vi "Python DENSO Communication.vi"() -> ()   [LabVIEW 2022 SP3]
uses:
  <vilib>/ImagingLab/Denso Robotics Library/_Private/Controls/drl_Variable T.ctl
  <vilib>/ImagingLab/Denso Robotics Library/_Private/Controls/drl_Motion parameters.ctl
  <vilib>/ImagingLab/Denso Robotics Library/_Private/Controls/drl_Interpolation.ctl
  <vilib>/ImagingLab/Denso Robotics Library/_Private/Controls/drl_Pass motion.ctl
  <vilib>/ImagingLab/Denso Robotics Library/_Private/Controls/drl_Move option.ctl
  <vilib>/ImagingLab/Denso Robotics Library/_Private/Controls/drl_Robot Coordinates.ctl
  <vilib>/ImagingLab/Denso Robotics Library/_Private/Controls/drl_Variable J.ctl
  <vilib>/Utility/error.llb/DialogType.ctl
  <vilib>/addons/zeromq/socket_type.ctl
  <vilib>/ImagingLab/Denso Robotics Library/_Private/Controls/drl_Robot Session.ctl
  <vilib>/ImagingLab/Denso Robotics Library/_Private/Controls/drl_Open Data.ctl
  <vilib>/ImagingLab/Denso Robotics Library/_Private/Controls/drl_Controller_IP Address.ctl
  <vilib>/ImagingLab/Denso Robotics Library/_Private/Controls/drl_Robot type.ctl
  <vilib>/ImagingLab/Denso Robotics Library/_Private/Controls/drl_controller_type.ctl
  <vilib>/ImagingLab/Denso Robotics Library/_Private/Controls/drl_Robot Motor status.ctl
  <vilib>/ImagingLab/Denso Robotics Library/_Private/Controls/drl_RobSlave actions.ctl
  <vilib>/ImagingLab/Denso Robotics Library/_Private/Controls/drl_Get_Set.ctl
  <vilib>/ImagingLab/Denso Robotics Library/_Private/Controls/drl_TOOL.ctl
  <vilib>/ImagingLab/Denso Robotics Library/_Public/SubVIs/drl_Robot Move_TRANS.vi
  <vilib>/ImagingLab/Denso Robotics Library/_Public/SubVIs/drl_Robot Move_JOINT.vi
  <vilib>/ImagingLab/Denso Robotics Library/_Public/SubVIs/drl_Robot Move_CARTESIAN.vi
  <vilib>/ImagingLab/Denso Robotics Library/_Public/SubVIs/drl_Get_Robot Angle_J.vi
  <vilib>/ImagingLab/Denso Robotics Library/_Public/SubVIs/drl_Get_Robot Position_P.vi
  <vilib>/ImagingLab/Denso Robotics Library/_Public/SubVIs/drl_Get_Robot Trans_T.vi
  <vilib>/addons/zeromq/zmq_context.lvclass
  <vilib>/addons/zeromq/zmq_socket.lvclass
  <vilib>/addons/zeromq/zeromq.lvlib
  <vilib>/ImagingLab/Denso Robotics Library/DensoRoboticsLibrary.lvlib
panel:
  in  "stop":bool
  in  "Communication port":string="5555"
  out "Motion parameters J":T1
  out "Position J":T5 {"Axis 6" format="%.4f"; "Axis 5" format="%.4f"; "Axis 4" format="%.4f"; "Axis 3" format="%.4f"; "Axis 2" format="%.4f"; "Axis 1" format="%.4f"}
  out "Motion parameters C":T1
  out "Position C":T6 {"X" format="%.4f"; "Y" format="%.4f"; "Z" format="%.4f"; "Rx" format="%.4f"; "Ry" format="%.4f"; "Rz" format="%.4f"}
  out "Motion parameters T":T1
  out "Position T":T7 {"Az" format="%.4f"; "Ay" format="%.4f"; "Ax" format="%.4f"; "Oz" format="%.4f"; "Oy" format="%.4f"; "Ox" format="%.4f"; "Z" format="%.4f"; "Y" format="%.4f"; "X" format="%.4f"}
  out "Message history":string[][](array[string])
  out "Python message string - data":string
  out "Python message string - command":string
  out "Python message string":string
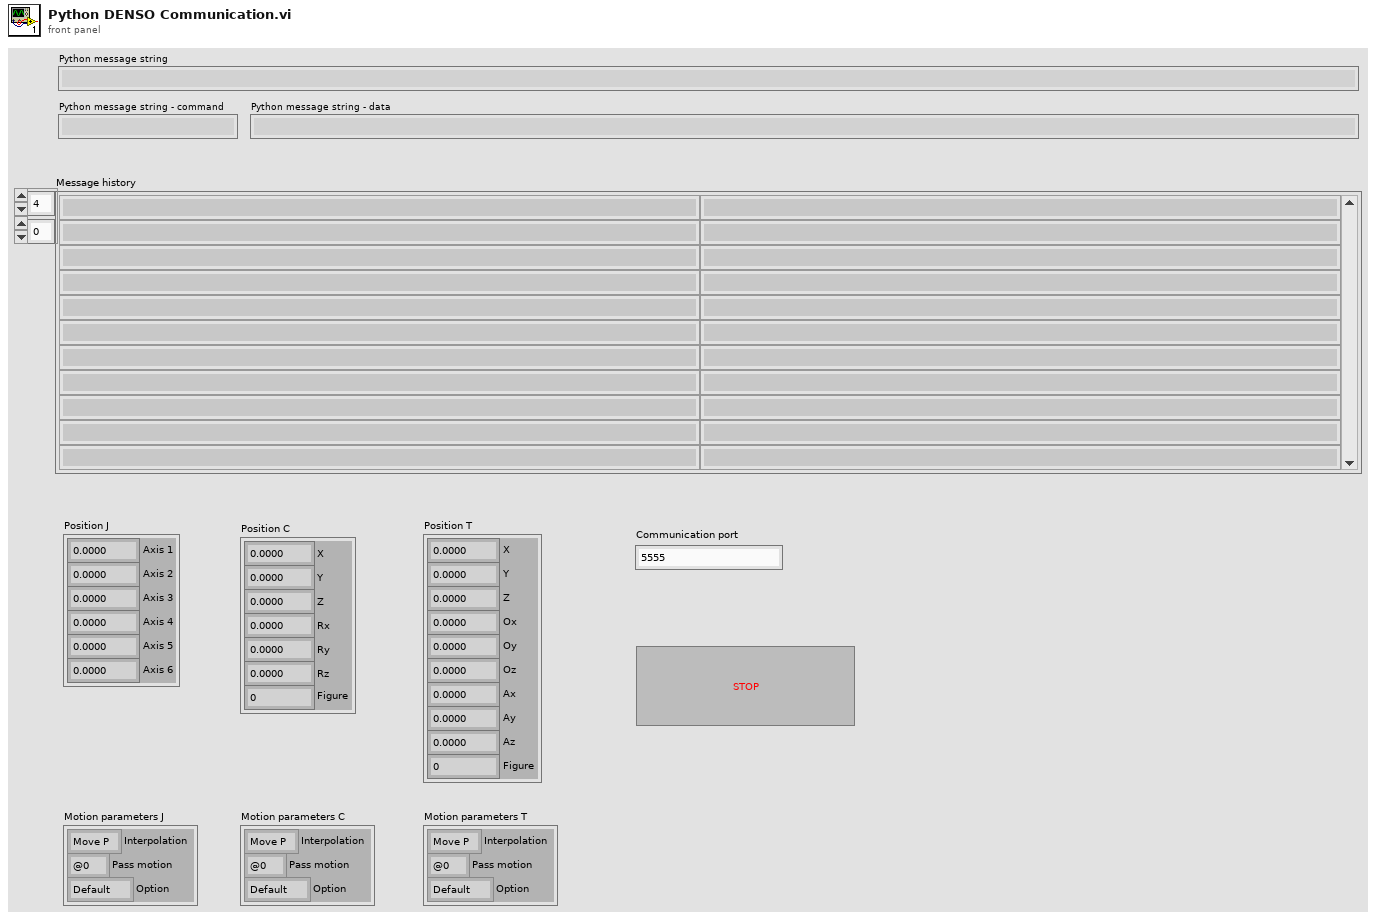
[diagram p1: front panel]
types:
  T1 = typedef "DensoRoboticsLibrary.lvlib/drl_Motion parameters.ctl" = cluster{"Interpolation":T2, "Pass motion":T3, "Option":T4}
  T2 = typedef "DensoRoboticsLibrary.lvlib/drl_Interpolation.ctl" = enum16{"Move P", "Move L"}
  T3 = typedef "DensoRoboticsLibrary.lvlib/drl_Pass motion.ctl" = enum16{"@0", "@P", "@E"}
  T4 = typedef "DensoRoboticsLibrary.lvlib/drl_Move option.ctl" = enum16{"Default", "Next"}
  T5 = typedef "DensoRoboticsLibrary.lvlib/drl_Variable J.ctl" = cluster{"Axis 1":sgl, "Axis 2":sgl, "Axis 3":sgl, "Axis 4":sgl, "Axis 5":sgl, "Axis 6":sgl}
  T6 = typedef "DensoRoboticsLibrary.lvlib/drl_Robot Coordinates.ctl" = cluster{"X":dbl, "Y":dbl, "Z":dbl, "Rx":dbl, "Ry":dbl, "Rz":dbl, "Figure":dbl}
  T7 = typedef "DensoRoboticsLibrary.lvlib/drl_Variable T.ctl" = cluster{"X":sgl, "Y":sgl, "Z":sgl, "Ox":sgl, "Oy":sgl, "Oz":sgl, "Ax":sgl, "Ay":sgl, "Az":sgl, "Figure":sgl}
  T8 = typedef "zeromq.lvlib/socket_type.ctl" = enum8{"ZMQ_PAIR", "ZMQ_PUB", "ZMQ_SUB", "ZMQ_REQ", "ZMQ_REP", "ZMQ_DEALER", "ZMQ_ROUTER", "ZMQ_PULL", "ZMQ_PUSH", "ZMQ_XPUB", "ZMQ_XSUB", "ZMQ_STREAM", "ZMQ_SERVER", "ZMQ_CLIENT", "ZMQ_RADIO", "ZMQ_DISH", "ZMQ_GATHER", "ZMQ_SCATTER", "ZMQ_DGRAM"}
  T9 = typedef "DensoRoboticsLibrary.lvlib/drl_Robot Session.ctl" = string
  T10 = typedef "DensoRoboticsLibrary.lvlib/drl_Open Data.ctl" = cluster{"controller IP address":T11, "robot type":T12, "controller type":T13}
  T11 = typedef "DensoRoboticsLibrary.lvlib/drl_Controller_IP Address.ctl" = string
  T12 = typedef "DensoRoboticsLibrary.lvlib/drl_Robot type.ctl" = enum16{"6 axes", "5 axes", "4 axes"}
  T13 = typedef "DensoRoboticsLibrary.lvlib/drl_controller_type.ctl" = enum16{"RC7", "RC8"}
  T14 = typedef "DensoRoboticsLibrary.lvlib/drl_Robot Motor status.ctl" = enum16{"Motor OFF", "Motor ON"}
  T15 = typedef "DensoRoboticsLibrary.lvlib/drl_RobSlave actions.ctl" = enum16{"Start", "Stop"}
  T16 = typedef "DensoRoboticsLibrary.lvlib/drl_Get_Set.ctl" = enum16{"Get", "Set"}
  T17 = typedef "DensoRoboticsLibrary.lvlib/drl_TOOL.ctl" = cluster{"X":sgl, "Y":sgl, "Z":sgl, "RX":sgl, "RY":sgl, "RZ":sgl}
  T18 = typedef "DialogType.ctl" = u16
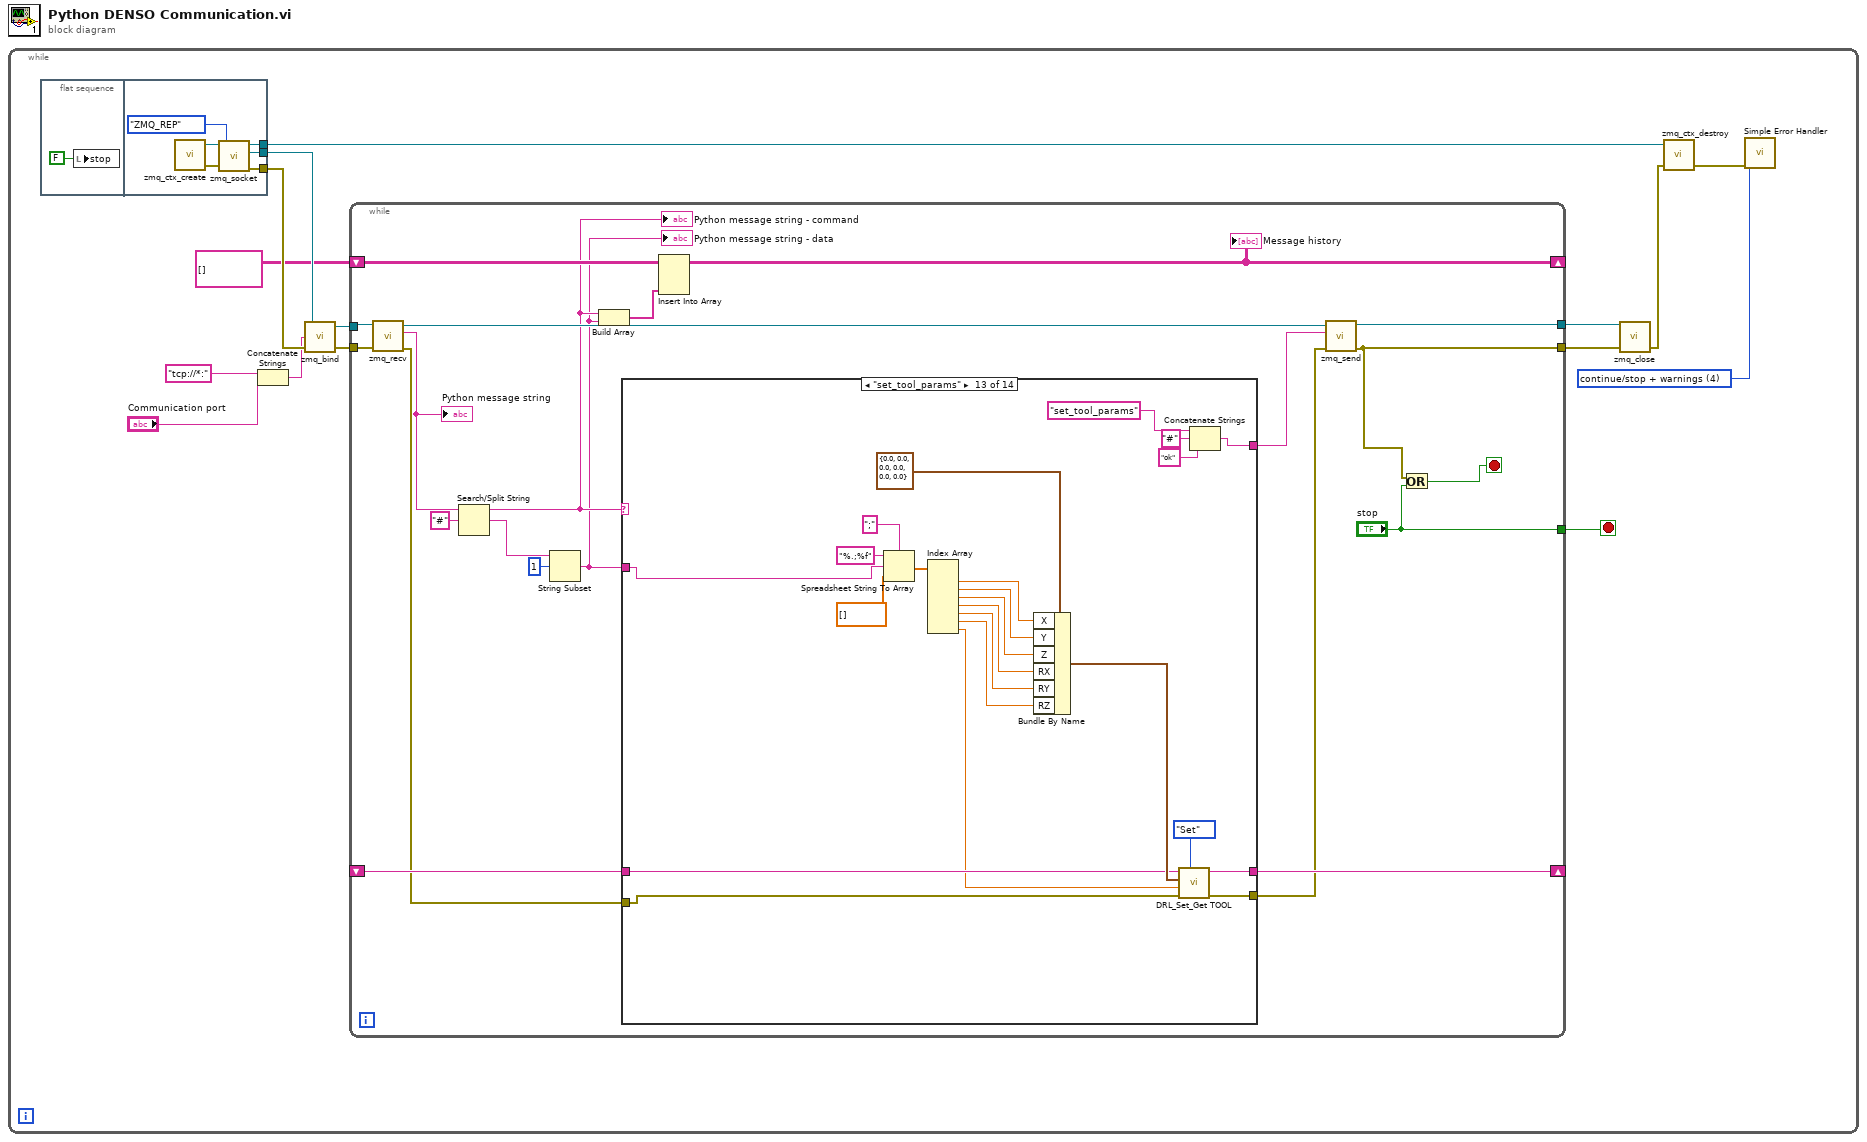
[diagram p0: block diagram]
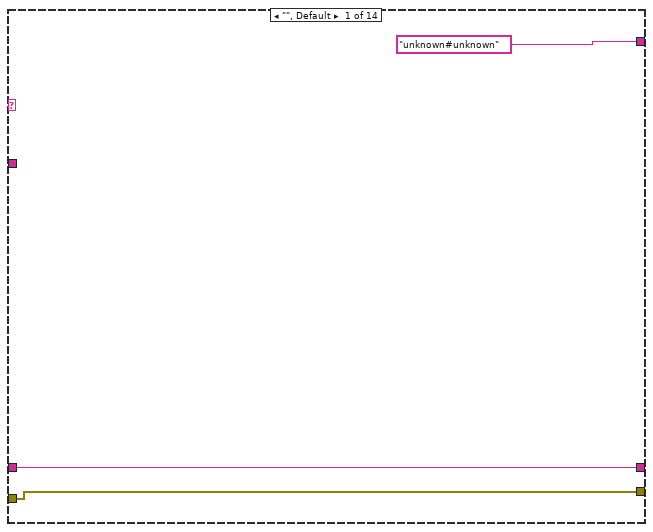
[diagram p2: hidden frame]
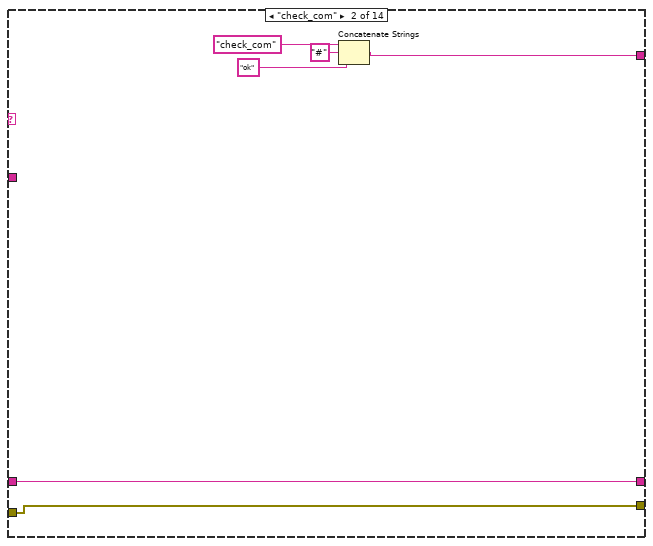
[diagram p3: hidden frame]
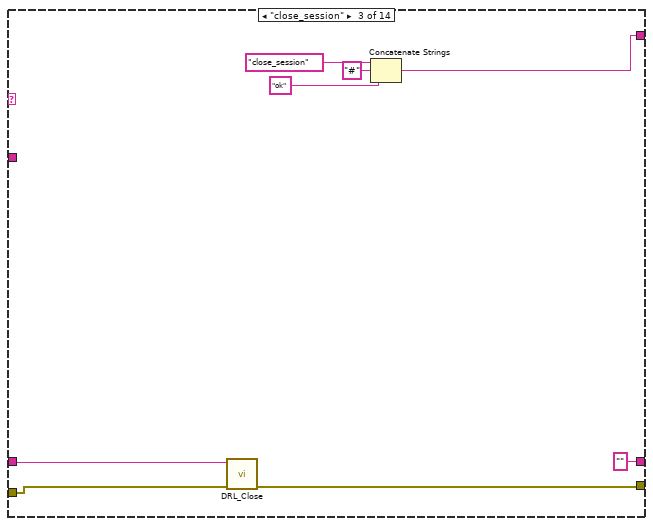
[diagram p4: hidden frame]
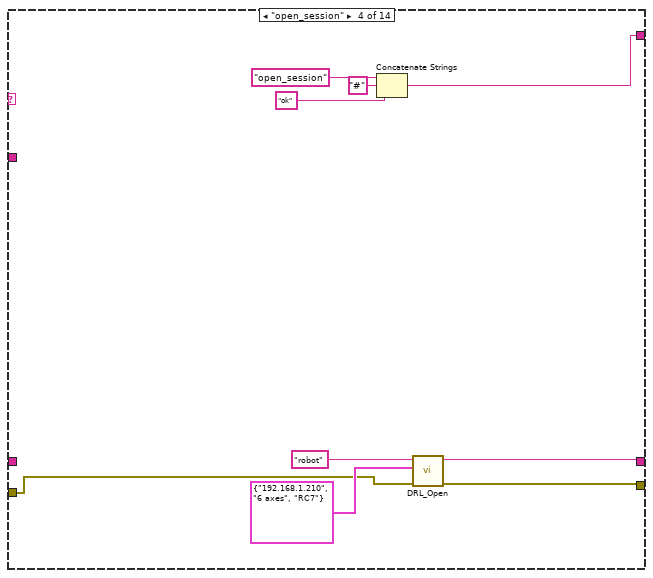
[diagram p5: hidden frame]
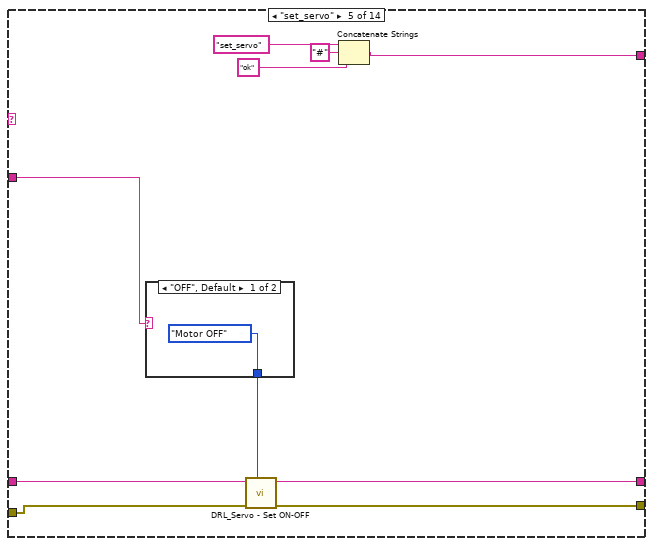
[diagram p6: hidden frame]
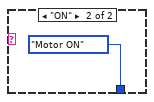
[diagram p7: hidden frame]
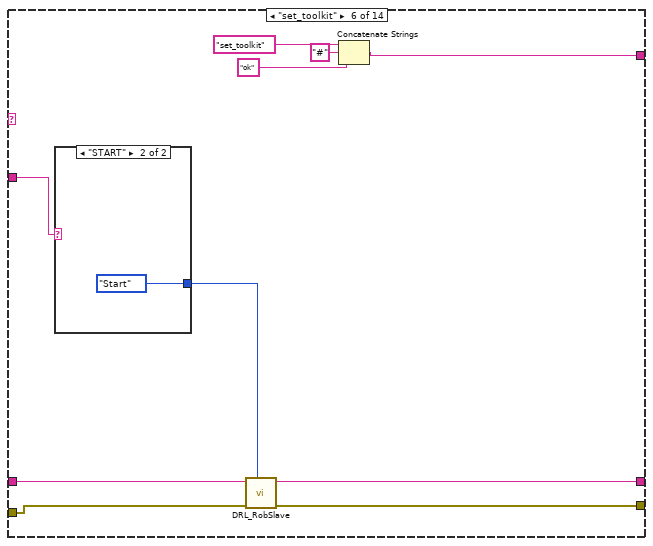
[diagram p8: hidden frame]
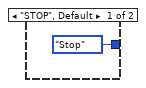
[diagram p9: hidden frame]
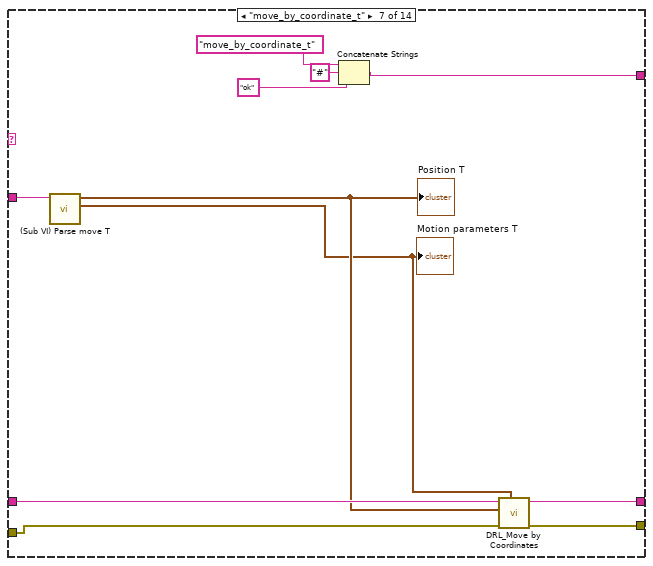
[diagram p10: hidden frame]
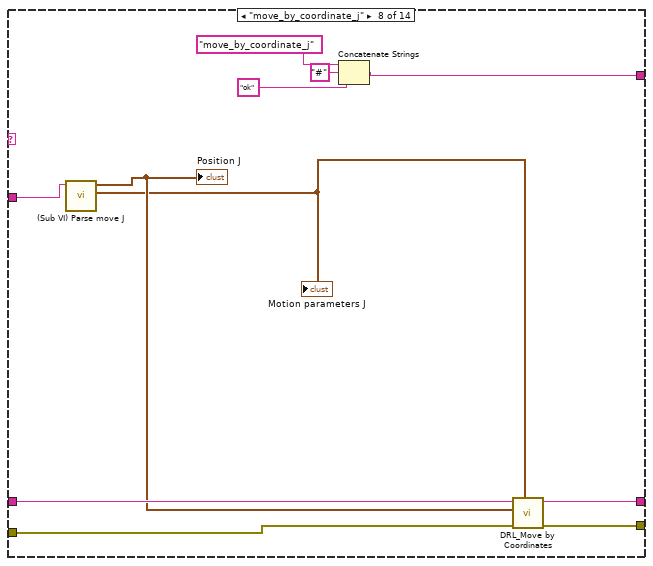
[diagram p11: hidden frame]
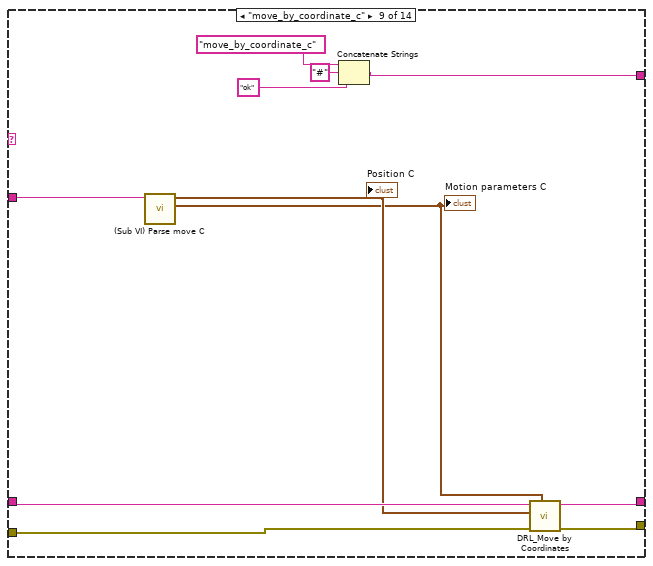
[diagram p12: hidden frame]
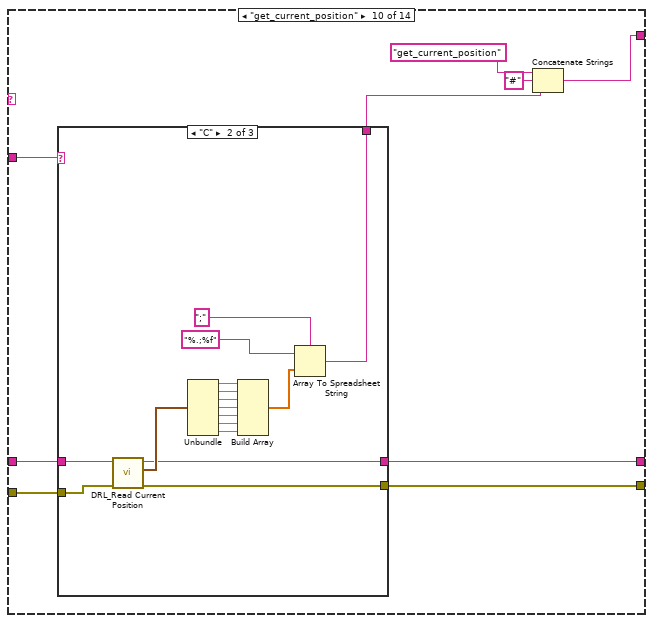
[diagram p13: hidden frame]
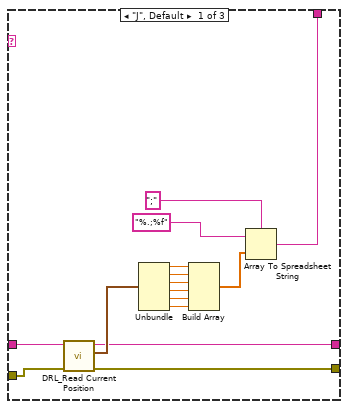
[diagram p14: hidden frame]
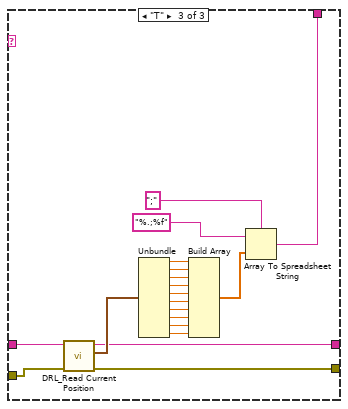
[diagram p15: hidden frame]
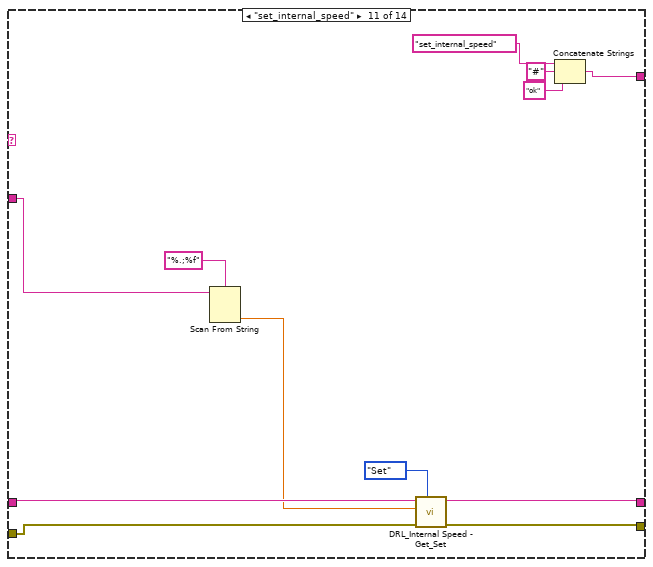
[diagram p16: hidden frame]
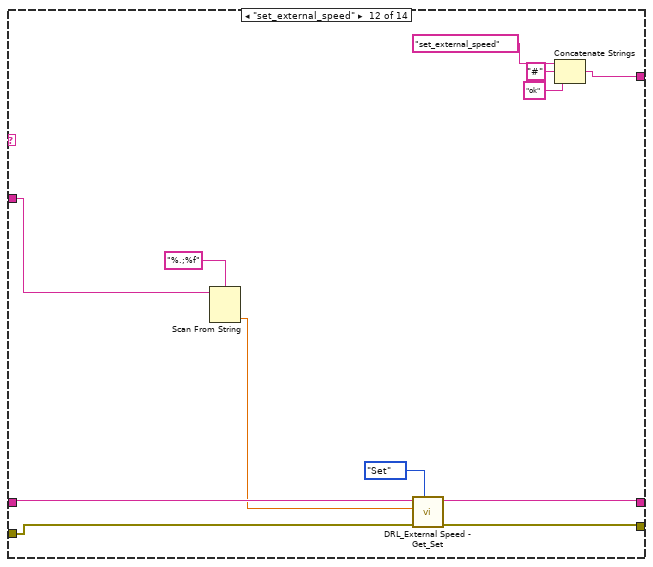
[diagram p17: hidden frame]
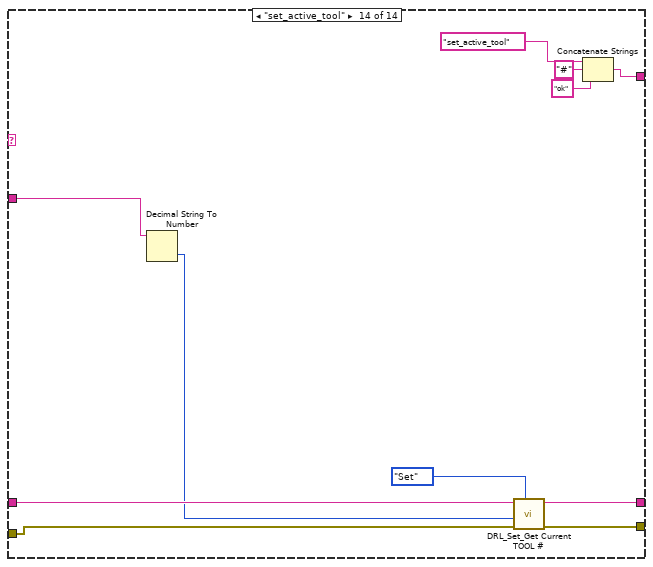
[diagram p18: hidden frame]
diagram:
  n1 = while {
    stop <- w1 stop-if-true
    w2 = T18 4 items=["no dialog", "OK message", "continue or stop message", "OK message + warnings", "continue/stop + warnings"] ("type of dialog (OK msg:1)")
    n2 = flat-sequence {
      tunnel: [w22] -> w15
      tunnel: [w21] -> w14
      tunnel: [w17] -> w8
      frame #0 {
        n3 = local write "stop"(FALSE ("stop")) -> ()
      }
      frame #1 {
        n4 = call <vilib>:"zmq_ctx_create.vi"() -> ("error out"=w20:errorcluster, "context out"=w19:refnum<class "zmq_context.lvclass">)  [unwired: 4 in]
        n5 = call <vilib>:"zmq_socket.vi"("error in"=w20, "socket type"=socket_type."ZMQ_REP", "context in"=w19) -> ("error out"=w22:errorcluster, "socket out"=w21:refnum<class "zmq_socket.lvclass">, "context out"=w17:refnum<class "zmq_context.lvclass">)  [unwired: 2 in]
      }
    }
    n6 = Concatenate Strings("tcp://*:" ("endpoint"), "Communication port") -> (w4:string)
    n7 = call <vilib>:"zmq_bind.vi"("error in"=w15, "endpoint"=w4, "socket in"=w14) -> ("error out"=w12:errorcluster, "socket out"=w13:refnum<class "zmq_socket.lvclass">)  [unwired: 1 in]
    n8 = while {
      tunnel: w13 -> [w42]
      tunnel: w12 -> [w43]
      tunnel: [w25] -> w11
      tunnel: [w40] -> w10
      shift-right: [w33] -> _
      shift-left: string[][] [] -> [w34]
      shift-right: [w29] -> _
      shift-left: _ -> [w28]
      tunnel: ["stop"] -> w1
      stop <- w24 stop-if-true
      n9 = call <vilib>:"zmq_recv.vi"("error in"=w43, "socket in"=w42) -> ("error out"=w27:errorcluster, "data"=w39:string, "socket out"=w41:refnum<class "zmq_socket.lvclass">)  [unwired: 3 in, 2 out]
      "Python message string" <- w39
      n10 = Search/Split String(string=w39, search string/char (-)="#") -> (substring before match=w32:string, match + rest of string=w37:string)  [unwired: 1 in, 1 out]
      "Python message string - command" <- w32
      n11 = String Subset(string=w37, offset (0)=1) -> (substring=w31:string)  [unwired: 1 in]
      "Python message string - data" <- w31
      n12 = Build Array(w32, w31) -> (w30:string[])
      n13 = case shown="\"set_tool_params\"" w32 {
        tunnel: w31 -> [_ _ _ _ w72 w85 w100 w111 w122 w135 w193 w205 w210 w240]
        tunnel: ["unknown#unknown" w49 w55 w63 w76 w88 w101 w112 w123 w131 w194 w206 w213 w235] -> w35
        tunnel: [w45 w48 T9 "" ("robot session*") w67 w73 w86 w96 w107 w118 w130 w188 w202 w219 w241] -> w29
        tunnel: w28 -> [w45 w48 w60 _ w74 w87 w99 w110 w121 w134 w191 w203 w218 w242]
        tunnel: w27 -> [w44 w47 w54 w62 w71 w83 w95 w106 w116 w128 w187 w199 w212 w234]
        tunnel: [w44 w47 w53 w61 w70 w82 w94 w105 w117 w127 w186 w198 w211 w233] -> w26
        frame "", Default {
        }
        frame "check_com" {
          n14 = Concatenate Strings("check_com", "#" ("string"), "ok" ("string")) -> (w49:string)
        }
        frame "close_session" {
          n15 = call <vilib>:"DRL_Close.vi"("error in (no error)"=w54, "robot session"=w60) -> ("error out"=w53:errorcluster)  [unwired: 9 in]
          n16 = Concatenate Strings("close_session", "#" ("string"), "ok" ("string")) -> (w55:string)
        }
        frame "open_session" {
          n17 = Concatenate Strings("open_session", "#" ("string"), "ok" ("string")) -> (w63:string)
          n18 = call <vilib>:"DRL_Open.vi"("error in (no error)"=w62, "connection settings"=T10 {"controller IP address"="192.168.1.210", "robot type"=enum."6 axes", "controller type"=enum."RC7"}, "robot session"=T9 "robot") -> ("error out"=w61:errorcluster, "robot session*"=w67:T9)  [unwired: 7 in]
        }
        frame "set_servo" {
          n19 = case shown="\"OFF\", Default" w72 {
            tunnel: [drl_Robot_Motor_status."Motor OFF" ("servo status") drl_Robot_Motor_status."Motor ON" ("servo status")] -> w75
            frame "OFF", Default {
            }
            frame "ON" {
            }
          }
          n20 = call <vilib>:"DRL_Servo - Set ON-OFF.vi"("servo status"=w75, "error in (no error)"=w71, "robot session"=w74) -> ("error out"=w70:errorcluster, "robot session*"=w73:T9)  [unwired: 7 in]
          n21 = Concatenate Strings("set_servo", "#" ("string"), "ok" ("string")) -> (w76:string)
        }
        frame "set_toolkit" {
          n22 = case shown="\"START\"" w85 {
            tunnel: [drl_RobSlave_actions."Stop" ("action") drl_RobSlave_actions."Start" ("action")] -> w84
            frame "STOP", Default {
            }
            frame "START" {
            }
          }
          n23 = call <vilib>:"DRL_RobSlave.vi"("action"=w84, "error in (no error)"=w83, "robot session"=w87) -> ("error out"=w82:errorcluster, "robot session*"=w86:T9)  [unwired: 7 in]
          n24 = Concatenate Strings("set_toolkit", "#" ("string"), "ok" ("string")) -> (w88:string)
        }
        frame "move_by_coordinate_t" {
          n25 = call "(Sub VI) Parse move T.vi"("data"=w100) -> ("Motion parameters"=w97:T1, "Position T"=w98:T7)  [unwired: 9 in]
          "Position T" <- w98
          "Motion parameters T" <- w97
          n26 = Concatenate Strings("move_by_coordinate_t", "#" ("string"), "ok" ("string")) -> (w101:string)
          n27 = call-poly <vilib>:"DRL_Move by Coordinates.vi"("motion parameters"=w97, "error in (no error)"=w95, "position T"=w98, "robot session"=w99) -> ("error out"=w94:errorcluster, "robot session*"=w96:T9)  [unwired: 6 in]
        }
        frame "move_by_coordinate_j" {
          n28 = call "(Sub VI) Parse move J.vi"("data"=w111) -> ("Motion parameters"=w108:T1, "Position J"=w109:T5)  [unwired: 9 in]
          "Position J" <- w109
          "Motion parameters J" <- w108
          n29 = Concatenate Strings("move_by_coordinate_j", "#" ("string"), "ok" ("string")) -> (w112:string)
          n30 = call-poly <vilib>:"DRL_Move by Coordinates.vi"("motion parameters"=w108, "error in (no error)"=w106, "position J"=w109, "robot session"=w110) -> ("error out"=w105:errorcluster, "robot session*"=w107:T9)  [unwired: 6 in]
        }
        frame "move_by_coordinate_c" {
          n31 = call "(Sub VI) Parse move C.vi"("data"=w122) -> ("Motion parameters"=w119:T1, "Position C"=w120:T6)  [unwired: 9 in]
          "Position C" <- w120
          "Motion parameters C" <- w119
          n32 = Concatenate Strings("move_by_coordinate_c", "#" ("string"), "ok" ("string")) -> (w123:string)
          n33 = call-poly <vilib>:"DRL_Move by Coordinates.vi"("motion parameters"=w119, "error in (no error)"=w116, "robot coordinates"=w120, "robot session"=w121) -> ("error out"=w117:errorcluster, "robot session*"=w118:T9)  [unwired: 6 in]
        }
        frame "get_current_position" {
          n34 = case shown="\"C\"" w135 {
            tunnel: w134 -> [w150 w166 w185]
            tunnel: [w148 w164 w183] -> w130
            tunnel: [w138 w154 w173] -> w129
            tunnel: w128 -> [w137 w152 w168]
            tunnel: [w136 w151 w167] -> w127
            frame "J", Default {
              n35 = call-poly <vilib>:"DRL_Read Current Position.vi"("error in (no error)"=w137, "robot session"=w150) -> ("error out"=w136:errorcluster, "position J"=w149:T5, "robot session*"=w148:T9)  [unwired: 7 in]
              n36 = Unbundle(w149) -> ("Axis 1"=w145:sgl, "Axis 2"=w144:sgl, "Axis 3"=w143:sgl, "Axis 4"=w142:sgl, "Axis 5"=w141:sgl, "Axis 6"=w140:sgl)
              n37 = Build Array(w145, w144, w143, w142, w141, w140) -> (w139:sgl[])
              n38 = Array To Spreadsheet String(delimiter (Tab)=";", array=w139, 3:"%.;%f" ("format string")) -> (spreadsheet string=w138:string)
            }
            frame "C" {
              n39 = call-poly <vilib>:"DRL_Read Current Position.vi"("error in (no error)"=w152, "robot session"=w166) -> ("error out"=w151:errorcluster, "position P"=w165:T6, "robot session*"=w164:T9)  [unwired: 7 in]
              n40 = Unbundle(w165) -> ("X"=w161:dbl, "Y"=w160:dbl, "Z"=w159:dbl, "Rx"=w158:dbl, "Ry"=w157:dbl, "Rz"=w156:dbl, "Figure"=w153:dbl)
              n41 = Build Array(w161, w160, w159, w158, w157, w156, w153) -> (w155:dbl[])
              n42 = Array To Spreadsheet String(delimiter (Tab)=";", array=w155, 3:"%.;%f" ("format string")) -> (spreadsheet string=w154:string)
            }
            frame "T" {
              n43 = call-poly <vilib>:"DRL_Read Current Position.vi"("error in (no error)"=w168, "robot session"=w185) -> ("error out"=w167:errorcluster, "position T"=w184:T7, "robot session*"=w183:T9)  [unwired: 7 in]
              n44 = Unbundle(w184) -> ("X"=w180:sgl, "Y"=w179:sgl, "Z"=w178:sgl, "Ox"=w177:sgl, "Oy"=w176:sgl, "Oz"=w175:sgl, "Ax"=w172:sgl, "Ay"=w171:sgl, "Az"=w170:sgl, "Figure"=w169:sgl)
              n45 = Build Array(w180, w179, w178, w177, w176, w175, w172, w171, w170, w169) -> (w174:sgl[])
              n46 = Array To Spreadsheet String(delimiter (Tab)=";", array=w174, 3:"%.;%f" ("format string")) -> (spreadsheet string=w173:string)
            }
          }
          n47 = Concatenate Strings("get_current_position", "#" ("string"), w129) -> (w131:string)
        }
        frame "set_internal_speed" {
          n48 = Scan From String(format string="%.;%f", input string=w193) -> (output 1=w190:dbl)  [unwired: 3 in, 3 out]
          n49 = call <vilib>:"DRL_Internal Speed - Get_Set.vi"("action"=drl_Get_Set."Set", "error in (no error)"=w187, "int speed in"=w190, "robot session"=w191) -> ("error out"=w186:errorcluster, "robot session*"=w188:T9)  [unwired: 5 in, 1 out]
          n50 = Concatenate Strings("set_internal_speed", "#" ("string"), "ok" ("string")) -> (w194:string)
        }
        frame "set_external_speed" {
          n51 = Scan From String(format string="%.;%f", input string=w205) -> (output 1=w200:dbl)  [unwired: 3 in, 3 out]
          n52 = call <vilib>:"DRL_External Speed - Get_Set.vi"("action"=drl_Get_Set."Set", "error in (no error)"=w199, "ext speed in"=w200, "robot session"=w203) -> ("error out"=w198:errorcluster, "robot session*"=w202:T9)  [unwired: 5 in, 1 out]
          n53 = Concatenate Strings("set_external_speed", "#" ("string"), "ok" ("string")) -> (w206:string)
        }
        frame "set_tool_params" {
          n54 = Spreadsheet String To Array(delimiter (Tab)=";", format string="%.;%f", spreadsheet string=w210, array type (2D Dbl)=dbl[] []) -> (array=w227:dbl[])
          n55 = Index Array(array=w227) -> (element #1=w226:dbl, element #2=w225:dbl, element #3=w224:dbl, element #4=w223:dbl, element #5=w222:dbl, element #6=w221:dbl, element #7=w217:dbl)  [unwired: 7 in]
          n56 = Bundle By Name(cluster=T17 {"X"=0.0, "Y"=0.0, "Z"=0.0, "RX"=0.0, "RY"=0.0, "RZ"=0.0} ("Tool data"), "X"=w226, "Y"=w225, "Z"=w224, "RX"=w223, "RY"=w222, "RZ"=w221) -> (w220:T17)
          n57 = call <vilib>:"DRL_Set_Get TOOL.vi"("action"=drl_Get_Set."Set", "error in (no error)"=w212, "tool number"=w217, "tool data in"=w220, "robot session"=w218) -> ("error out"=w211:errorcluster, "robot session*"=w219:T9)  [unwired: 4 in, 1 out]
          n58 = Concatenate Strings("set_tool_params", "#" ("string"), "ok" ("string")) -> (w213:string)
        }
        frame "set_active_tool" {
          n59 = Decimal String To Number(string=w240) -> (number=w239:i32)  [unwired: 2 in, 1 out]
          n60 = call <vilib>:"DRL_Set_Get Current TOOL #.vi"("action"=drl_Get_Set."Set", "error in (no error)"=w234, "ID number in"=w239, "robot session"=w242) -> ("error out"=w233:errorcluster, "robot session"=w241:T9)  [unwired: 5 in, 1 out]
          n61 = Concatenate Strings("set_active_tool", "#" ("string"), "ok" ("string")) -> (w235:string)
        }
      }
      n62 = Insert Into Array(array=w34, new element=w30) -> (w33:string[][])  [unwired: 2 in]
      "Message history" <- w33
      n63 = call <vilib>:"zmq_send.vi"("error in"=w26, "data"=w35, "socket in"=w41) -> ("error out"=w25:errorcluster, "socket out"=w40:refnum<class "zmq_socket.lvclass">)  [unwired: 4 in]
      n64 = Or(x=w25, y="stop") -> (x .or. y?=w24:bool)
    }
    n65 = call <vilib>:"zmq_close.vi"("error in"=w11, "socket"=w10) -> ("error out"=w9:errorcluster)  [unwired: 3 in]
    n66 = call <vilib>:"zmq_ctx_destroy.vi"("error in"=w9, "context in"=w8) -> ("error out"=w3:errorcluster)  [unwired: 3 in]
    n67 = call <vilib>:"Simple Error Handler.vi"("type of dialog (OK msg:1)"=w2, "error in (no error)"=w3) -> ()  [unwired: 3 in, 5 out]
  }
